vi "winda.vi"() -> ()   [LabVIEW 2015]
panel:
  out "Cluster 2":T1
  in  "Exit":bool
  in  "Down":bool
  in  "Up":bool
  in  "Boolean 3":bool
  in  "Boolean 2":bool
  in  "Boolean":bool
  out "Cluster":T2
  out "Numeric 3":dbl
  in  "Numeric 2":dbl
  in  "Numeric":dbl
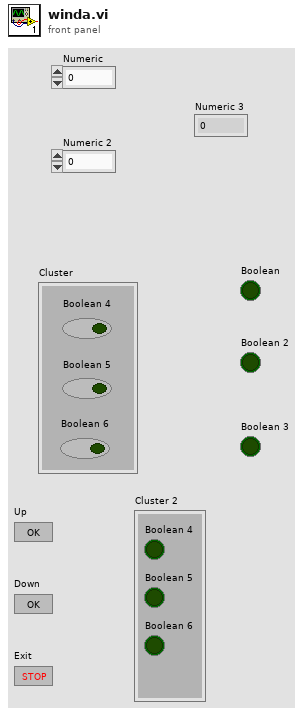
[diagram p1: front panel]
types:
  T1 = cluster{"Boolean 4":bool, "Boolean 5":bool, "Boolean 6":bool}
  T2 = cluster{"Boolean 4":bool, "Boolean 6":bool, "Boolean 5":bool}
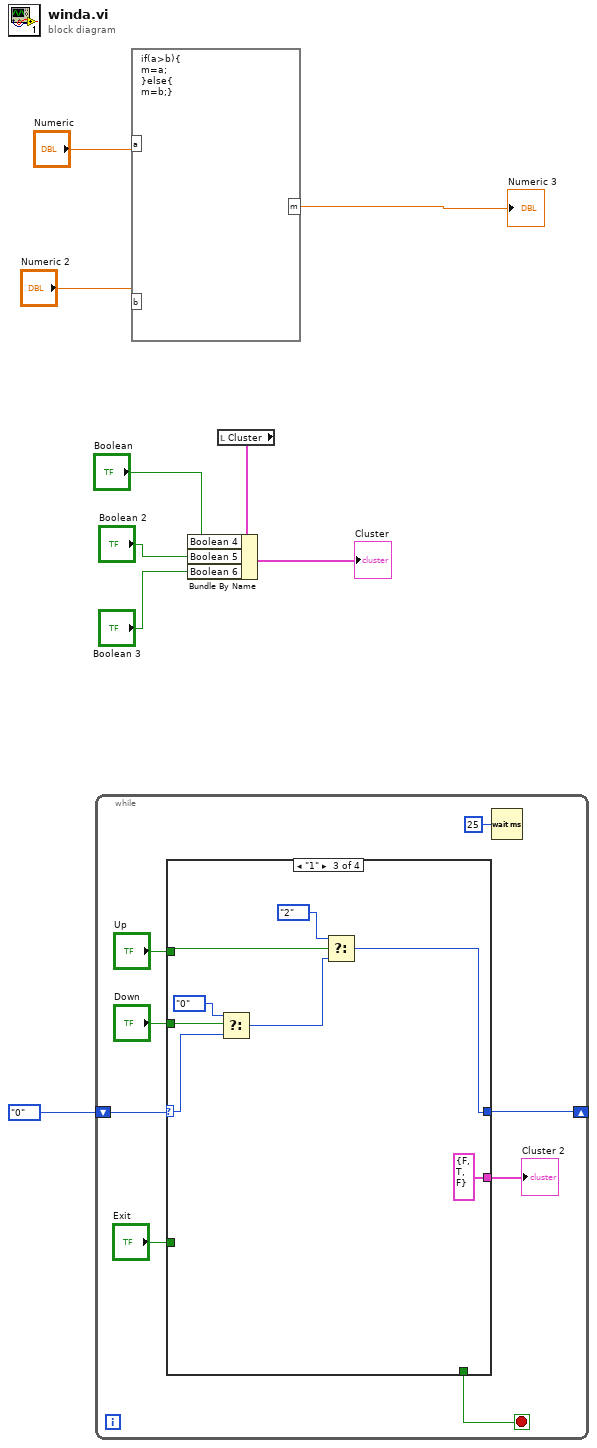
[diagram p0: block diagram]
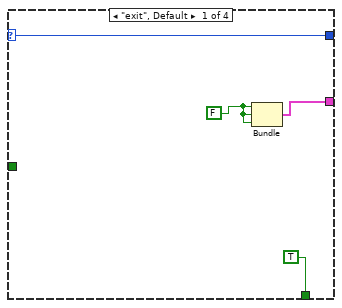
[diagram p2: hidden frame]
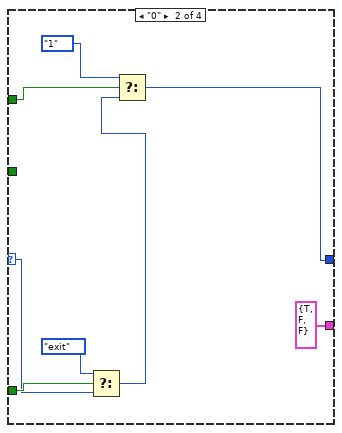
[diagram p3: hidden frame]
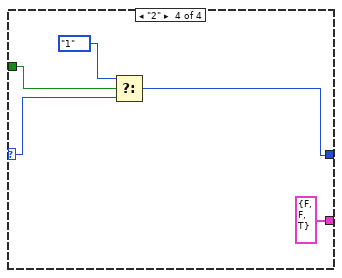
[diagram p4: hidden frame]
diagram:
  n1 = while {
    shift-right: [w10] -> _
    shift-left: enum16{"exit", "0", "1", "2"}."0" -> [w16]
    stop <- w15 stop-if-true
    n2 = case shown="\"1\"" w16 {
      selector: w16 -> [w18 w26 w35 w41]
      tunnel: [TRUE _ _ _] -> w15
      tunnel: [w19 cluster{bool, bool, bool} {TRUE, FALSE, FALSE} cluster{bool, bool, bool} {FALSE, TRUE, FALSE} cluster{bool, bool, bool} {FALSE, FALSE, TRUE}] -> w14
      tunnel: "Up" -> [_ w25 w36 _]
      tunnel: "Down" -> [_ _ w37 w42]
      tunnel: "Exit" -> [_ w28 _ _]
      tunnel: [w18 w23 w31 w39] -> w10
      frame "exit", Default {
        w20 = FALSE
        n3 = Bundle(w20, w20, w20) -> (w19:cluster{bool, bool, bool})  [unwired: 1 in]
      }
      frame "0" {
        n4 = Select(t=enum16{"exit", "0", "1", "2"}."exit", s=w28, f=w26) -> (s? t:f=w22:enum16{"exit", "0", "1", "2"})
        n5 = Select(t=enum16{"exit", "0", "1", "2"}."1", s=w25, f=w22) -> (s? t:f=w23:enum16{"exit", "0", "1", "2"})
      }
      frame "1" {
        n6 = Select(t=enum16{"exit", "0", "1", "2"}."0", s=w37, f=w35) -> (s? t:f=w32:enum16{"exit", "0", "1", "2"})
        n7 = Select(t=enum16{"exit", "0", "1", "2"}."2", s=w36, f=w32) -> (s? t:f=w31:enum16{"exit", "0", "1", "2"})
      }
      frame "2" {
        n8 = Select(t=enum16{"exit", "0", "1", "2"}."1", s=w42, f=w41) -> (s? t:f=w39:enum16{"exit", "0", "1", "2"})
      }
    }
    "Cluster 2" <- w14
    n9 = Wait (ms)(milliseconds to wait=u32 25) -> ()  [unwired: 1 out]
  }
  n10 = formula code="if(a>b){\nm=a;\n}else{\nm=b;}"("a"="Numeric", "b"="Numeric 2") -> ("m"=→"Numeric 3":dbl)
  n11 = local read "Cluster"() -> (w2:T2)
  n12 = Bundle By Name(cluster=w2, "Boolean 4"="Boolean", "Boolean 5"="Boolean 2", "Boolean 6"="Boolean 3") -> (→"Cluster":T2)
